vi "应用Y.vi"   [LabVIEW 2017]
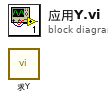
[diagram p0: block diagram]
diagram:
  n1 = call "求Y.vi"() -> ()  [unwired: 3 in, 1 out]
